vi "Stop Cooker.vi"(8 "error in (no error)":errorcluster, 11 "Ramp Cooker in":refnum<class "Ramp Cooker.lvclass">) -> (0 "error out":errorcluster, 2 "Finished?":bool, 3 "Ramp Cooker out":refnum<class "Ramp Cooker.lvclass">)   [LabVIEW 2024, in "Cooker Actor.lvlib" / "Ramp Cooker.lvclass"]
uses:
  Ramp Cooker.lvclass
  Ramp Cooker.lvclass/Ramp Cooker.ctl
  Cooker Actor/Cooker Actor.lvclass
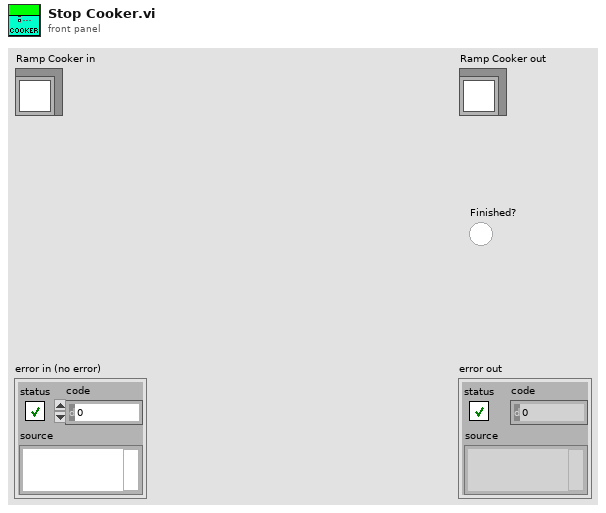
[diagram p1: front panel]
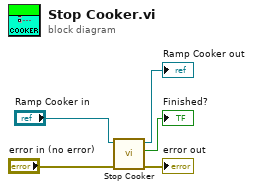
[diagram p0: block diagram]
diagram:
  n1 = call-parent "Stop Cooker.vi"("error in (no error)"="error in (no error)", "Cooker Actor in"="Ramp Cooker in") -> ("error out"=→"error out":errorcluster, "Finished?"=→"Finished?":bool, "Cooker Actor out"=→"Ramp Cooker out":refnum<class "Ramp Cooker.lvclass">)  [unwired: 7 in]
